vi "waitStatusSweepingStopped.vi"(8 "error in (no error)":errorcluster, 10 "time (s) [10 s]":dbl=10.0, 11 "Instrument.Lockin in":refnum<class "Instrument.Lockin.lvclass">) -> (0 "error out":errorcluster, 3 "Instrument.Lockin out":refnum<class "Instrument.Lockin.lvclass">)   [LabVIEW 2019, in "Instrument.Lockin.lvclass"]
uses:
  Instrument.Lockin.lvclass
  Instrument.DAQ/Typedefs/Get State-enum.ctl
  Instrument.DAQ/Instrument.DAQ.lvclass
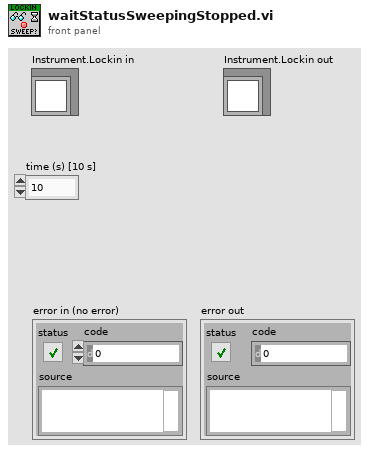
[diagram p1: front panel]
types:
  T1 = typedef "Instrument.DAQ.lvclass/Get State-enum.ctl" = enum16{"idle", "created", "started", "stopped", "sweeping"}
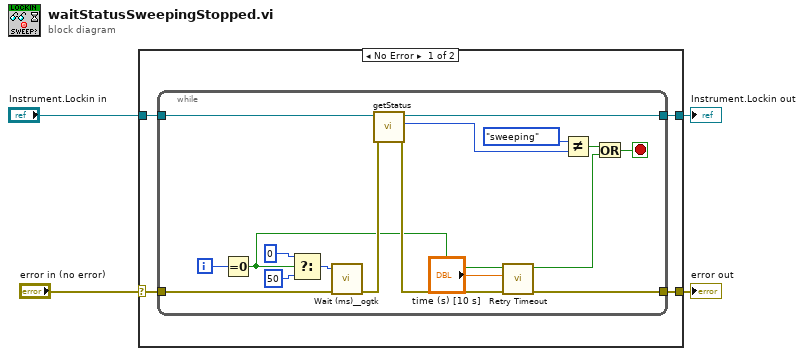
[diagram p0: block diagram]
diagram:
  n1 = case shown="No Error" "error in (no error)" {
    selector: "error in (no error)" -> [w5 w26]
    tunnel: [w8 w26] -> w4
    tunnel: [w7 w27] -> w3
    tunnel: "Instrument.Lockin in" -> [w6 w27]
    frame No Error {
      n2 = while {
        tunnel: w5 -> [w25]
        tunnel: [w14] -> w8
        tunnel: w6 -> [w20]
        tunnel: [w19] -> w7
        i -> [w12]
        stop <- w24 stop-if-true
        n3 = Equal To 0?(x=w12) -> (x = 0?=w11:bool)
        n4 = Select(t=u32 0, s=w11, f=u32 50 ("milliseconds to wait")) -> (s? t:f=w21:u32)
        n5 = call <userlib>:"Wait (ms)__ogtk.vi"("error in (no error)"=w25, "milliseconds to wait"=w21) -> ("error out"=w15:errorcluster)  [unwired: 8 in, 1 out]
        n6 = call "getStatus.vi"("error in (no error)"=w15, "Instrument.Lockin"=w20) -> ("error out"=w13:errorcluster, "Status"=w17:T1, "Instrument.Lockin"=w19:refnum<class "Instrument.Lockin.lvclass">)  [unwired: 7 in]
        n7 = call "Retry Timeout.vi"("error in (no error)"=w13, "time (s) [10 s]"="time (s) [10 s]", "reset"=w11) -> ("error out"=w14:errorcluster, "Timeout?"=w10:bool)  [unwired: 7 in]
        n8 = Not Equal?(x=Get_State-enum."sweeping" ("Status"), y=w17) -> (x != y?=w16:bool)
        n9 = Or(x=w16, y=w10) -> (x .or. y?=w24:bool)
      }
    }
    frame Error {
    }
  }
  "error out" <- w4
  "Instrument.Lockin out" <- w3
